vi "Ramp (2).vi"() -> ()   [LabVIEW 2016]
uses:
  controls/Enum.ctl
  <vilib>/rvi/errors/niLvFpgaAdjustHostInterfaceError.vi
  controls/FPGAVIreferenceTypeDef.ctl
  <vilib>/rvi/interface/nirviReadWriteControl/nirviReadWriteControl.xnode
  FPGA Bitfiles/qnmController797_usbRio80MHz_USB7856R80MHz.lvbitx
  <vilib>/rvi/interface/nirviMethod/nirviMethod.xnode
  <vilib>/regexp/Match Regular Expression.xnode
  Course Project/support/Message Queue/Message Queue.lvlib
  <vilib>/rvi/interface/nirviCloseFPGA/nirviCloseFPGA.xnode
  NiFpgaLv.dll
  <vilib>/rvi/errors/niLvFpgaMergeErrorWithErrorCode.vi
  <vilib>/FPGAPlugInAG/USB-7856R/niLvFpga_ReadFifo_USB-7856R.vi
  <vilib>/FPGAPlugInAG/USB-7856R/niLvFpga_Close_USB-7856R.vi
panel:
  in  "Display":T1(array[cluster])
  in  "Palet2":T2={"Save"=FALSE, "Delete"=FALSE, "Show 2"=TRUE}
  in  "Palet1":T2={"Save"=FALSE, "Delete"=FALSE, "Show 2"=TRUE}
  in  "ChannelDisplay2":u16(ring) items=["Height", "AI0 (error)"]
  in  "ChannelDisplay":u16(ring)=1 items=["Height", "AI0 (error)"]
  out "ForceCurves 2":cluster{dbl[], "Decimated Array":dbl[]}[](graph)
  out "ForceCurves":cluster{dbl[], "Decimated Array":dbl[]}[](graph)
  in  "Dec":u16=2 format="%#_3p"
  in  "recordClockDec":u16=100
  in  "SecureTip":T3 {"Sign" items=[">", "<"]; "Secure tip signal" items=["Vert. Deflection (V)", "Horiz. Deflection (V)", "Input 1", "Input 2"]; "Max-min-Tip" format="%#.2p"}
  in  "Curves 2":i32[](listbox)
  in  "Spectroscopy":enum32{"Spectroscopy"}(tab)
  in  "Reenable Feedback":bool=TRUE
  in  "LockSpeed":bool=TRUE
  in  "Direction":bool=TRUE
  in  "Fwd sweep":bool=TRUE
  in  "Parameters":T4={"Start"=-1e-06, "Distance"=1.1e-06, "Points"=1000.0, "Fwd"=5e-07, "Bwd"=5e-07, "Pause"=300.0} {"Pause" format="%#_3fms"; "Bwd" format="%_3pm/s"; "Distance" format="%#.3pm"; "Start" format="%#.3pm"; "Fwd" format="%_3pm/s"}
  out "Ramping?":bool
  in  "Bwd sweep":bool=TRUE
  in  "Output":enum16{"Z"}(ring)
  in  "Channels":i32[](listbox)=[0, 1]
  in  "Actions":T5={"Play"=FALSE, "Stop"=FALSE, "Loop"=FALSE, "Sweeps"=1.0} {"Sweeps" min=1.0 format="%#.0f"}
  in  "CalculateSlope":bool
  out "1/Slope":dbl format="%#_5pm/V"
  out "B":cluster{"Y":dbl, "X":dbl} {"X" format="%#_2p"; "Y" format="%#_2p"}
  out "A":cluster{"Y":dbl, "X":dbl} {"X" format="%#_2p"; "Y" format="%#_2p"}
  in  "Saving":T6={"#"=0, "Name"="", "Path"=path "C:/ForceCurves", "Autosave"=FALSE, "Save"=FALSE} {"#" format="%03.0f"}
  in  "Trigger Source":T7(ring)=enum."Relative Height"
  # "Secure tip"
  # "Spectroscopy"
  # "Trigger"
  # "Ramp"
  # "Cursors"
  # "-"
  # "+"
  # "Saving"
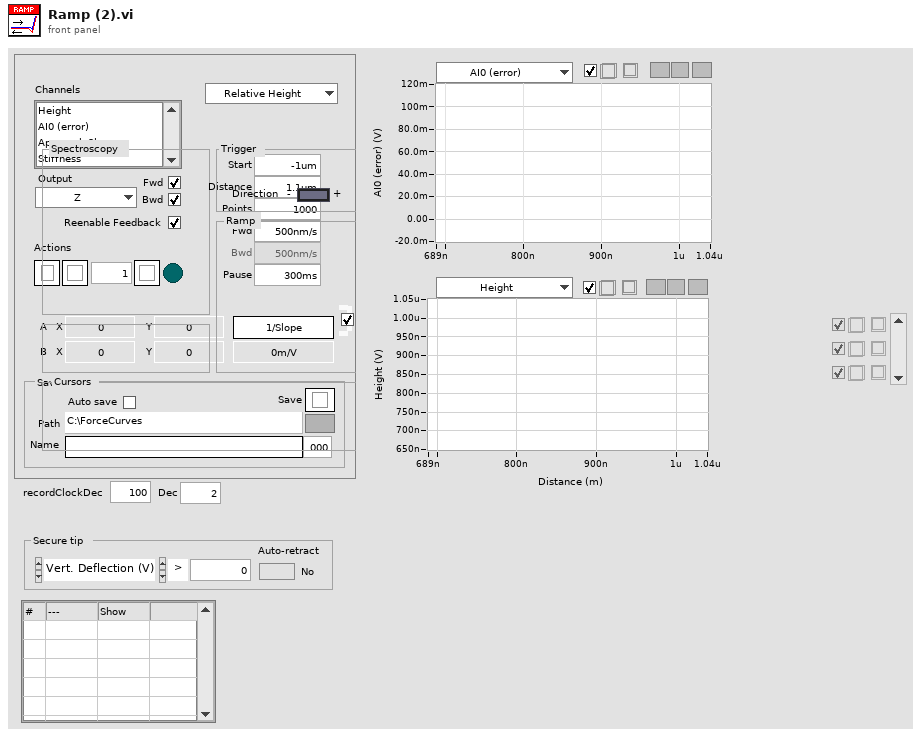
[diagram p1: front panel]
types:
  T1 = cluster{"Save":bool, "Delete":bool, "Show 2":bool}[]
  T2 = cluster{"Save":bool, "Delete":bool, "Show 2":bool}
  T3 = cluster{"Max-min-Tip":dbl, "Secure tip signal":u16, "Sign":u16, "Auto-retract":bool}
  T4 = cluster{"Start":dbl, "Distance":dbl, "Points":dbl, "Fwd":dbl, "Bwd":dbl, "Pause":dbl}
  T5 = cluster{"Play":bool, "Stop":bool, "Loop":bool, "Sweeps":dbl}
  T6 = cluster{"#":i64, "Name":string, "Path":path, "Autosave":bool, "Save":bool}
  T7 = enum16{"Absolute Height", "Process Variable", "External Source", "Relative Height"}
  T8 = typedef "Message Queue.lvlib/All Message Queues.ctl" = cluster{"IU":refnum<queue>}
  T9 = typedef "Enum.ctl" = enum16{"Init", "Read", "Write"}
  T10 = enum32{"Bad", "Idle", "Run top level", "Running"}
  T11 = enum8{"Enabled", "Disabled", "Disabled and Grayed Out"}
  T12 = enum16{"Absolute Height", "Process Variable", "External Source"}
  T13 = cluster{"Range Z":dbl, "Parameters":cluster{"Start":dbl, "Distance":dbl, "Points":dbl, "Fwd":dbl, "Bwd":dbl, "Pause":dbl}, "Trigger Source":enum16{"Absolute Height", "Process Variable", "External Source", "Relative Height"}}
  T14 = enum16{"open", "replace", "create", "open or create", "replace or create", "replace or create with confirmation"}
  T15 = cluster{"calibName":string[], "calibParameters":cluster{"Sensitivity":cluster{"Sens X":dbl, "Sens Y":dbl, "Sens Z":dbl}, "Range":cluster{"Range X":dbl, "Range Y":dbl, "Range Z":dbl}, "HV gain":cluster{"HV gain X":dbl, "HV gain Y":dbl, "HV gain Z":dbl}}[], "calibIndex":i32}
  T16 = cluster{"Sensitivity":cluster{"Sens X":dbl, "Sens Y":dbl, "Sens Z":dbl}, "Range":cluster{"Range X":dbl, "Range Y":dbl, "Range Z":dbl}, "HV gain":cluster{"HV gain X":dbl, "HV gain Y":dbl, "HV gain Z":dbl}}[]
  T17 = cluster{"Sensitivity":cluster{"Sens X":dbl, "Sens Y":dbl, "Sens Z":dbl}, "Range":cluster{"Range X":dbl, "Range Y":dbl, "Range Z":dbl}, "HV gain":cluster{"HV gain X":dbl, "HV gain Y":dbl, "HV gain Z":dbl}}
  T18 = typedef "FPGAVIreferenceTypeDef.ctl" = refnum<k20>
  T19 = typedef "FPGAVIreferenceTypeDefScanEngine.ctl" = refnum<k20>
  T20 = cluster{"enableManualMotion":bool, "doMove":bool, "integratorTarget":fxp<+/-,22,2>, "clocks":cluster{"inverseDecimation":fxp<+,22,0>, "decimation":u16, "waveSize":u16, "pixelDecimation":u16}}
  T21 = cluster{"rmp.p.resetStartPos":bool, "rmp.p.resetEndPos":bool}
  T22 = cluster{"rmp.p.downRate":fxp<+/-,22,-10>, "rmp.p.upRate":fxp<+/-,22,-10>, "rmp.p.startPos":fxp<+/-,24,2>, "rmp.p.clockDec":u16, "rmp.p.recordClockDec":u16, "rmp.p.enableHDTPointRecord":bool, "rmp.p.pull":bool}
  T23 = cluster{"rmp.triggerSource":u8, "rmp.p.triggerPositive":bool, "rmp.p.triggerLevel":fxp<+/-,24,16>}
  T24 = typedef "LVPointDoubleTypeDef.ctl" = cluster{"Cursor X":dbl, "Cursor Y":dbl}
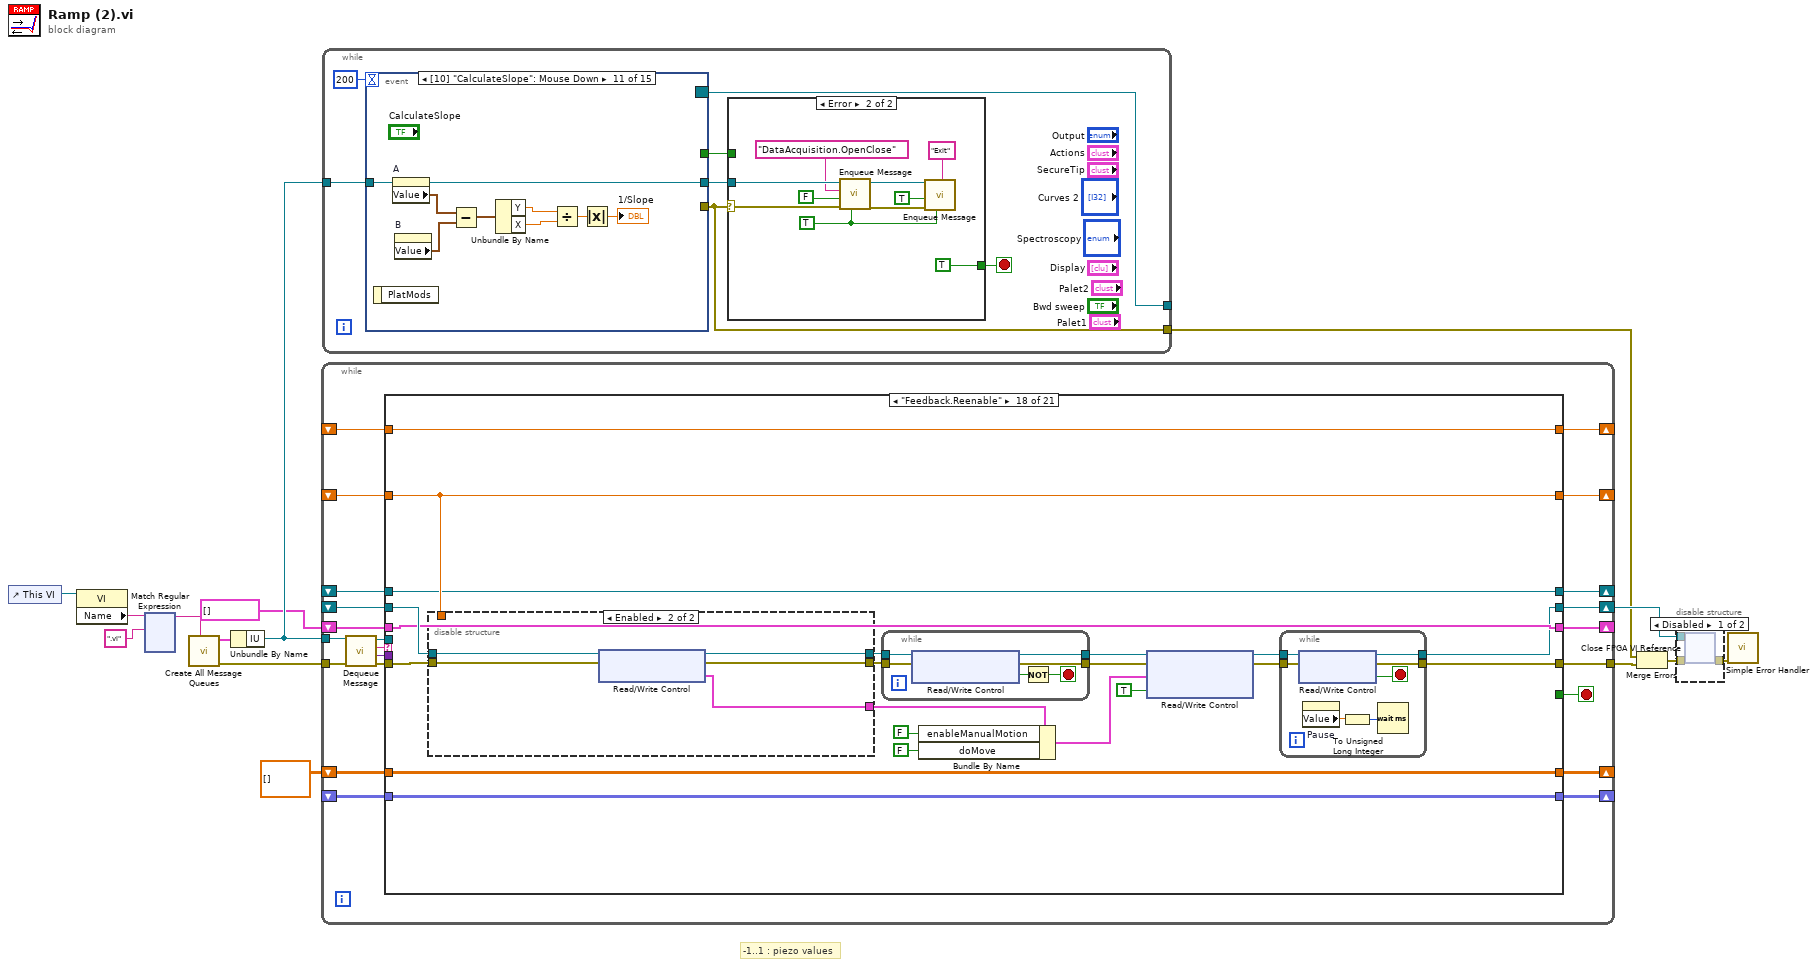
[diagram p0: block diagram]
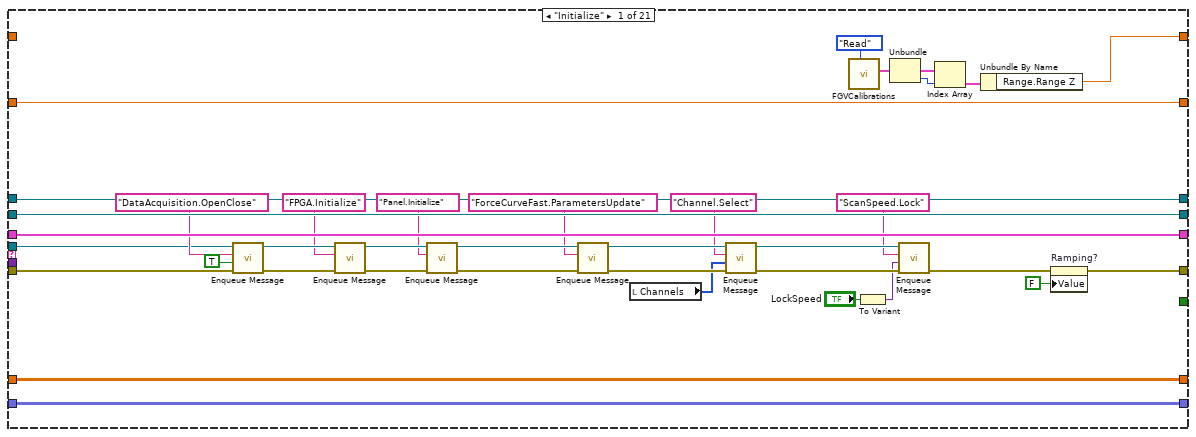
[diagram p3: hidden frame]
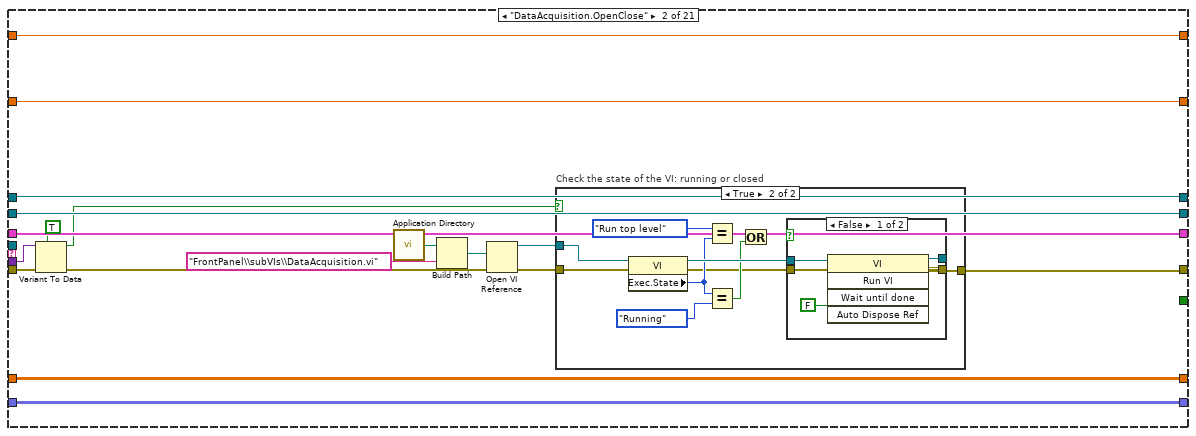
[diagram p4: hidden frame]
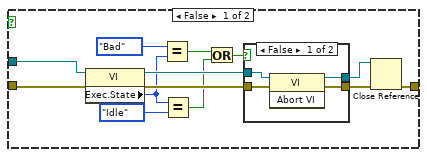
[diagram p5: hidden frame]
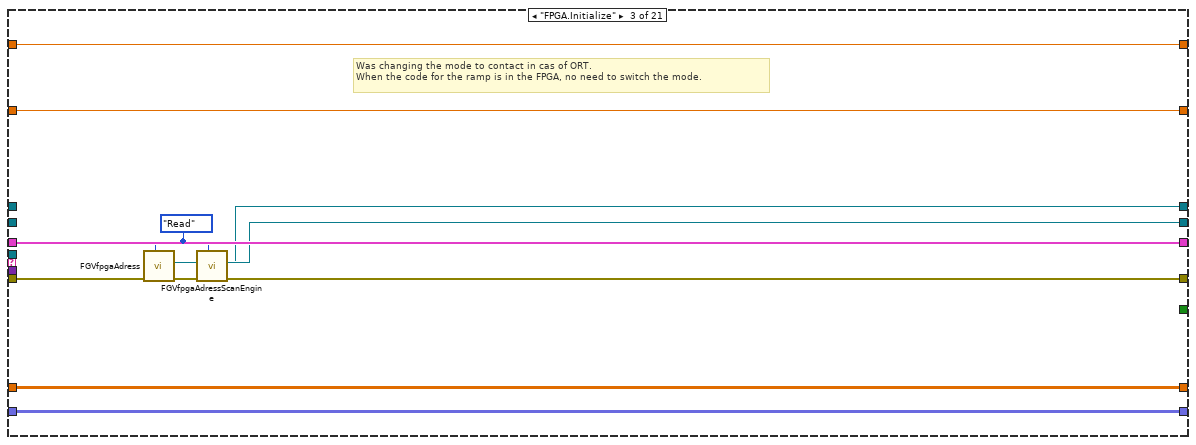
[diagram p8: hidden frame]
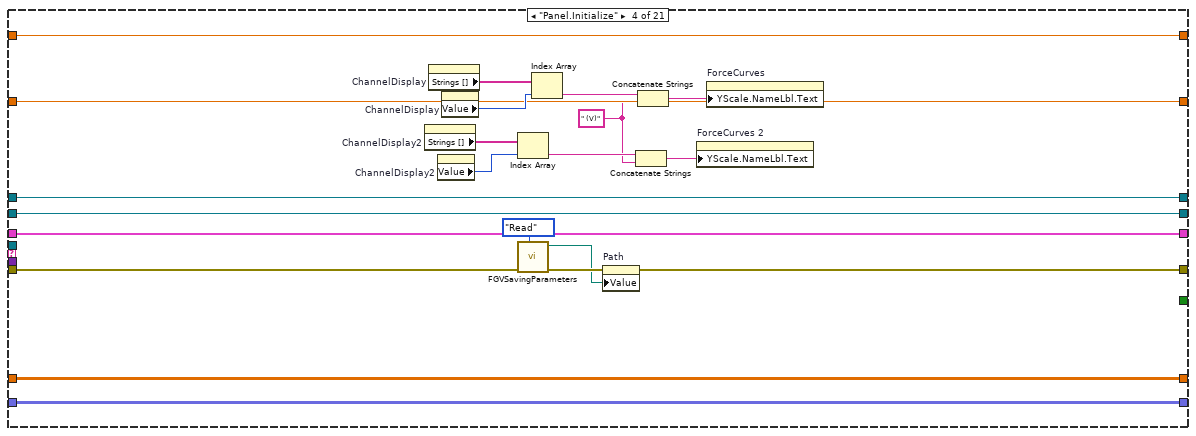
[diagram p9: hidden frame]
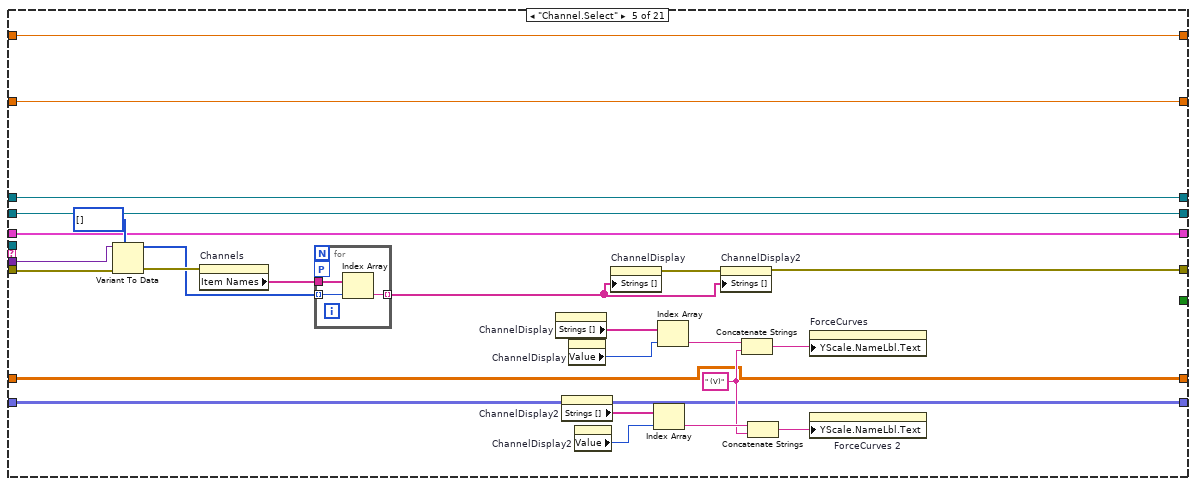
[diagram p10: hidden frame]
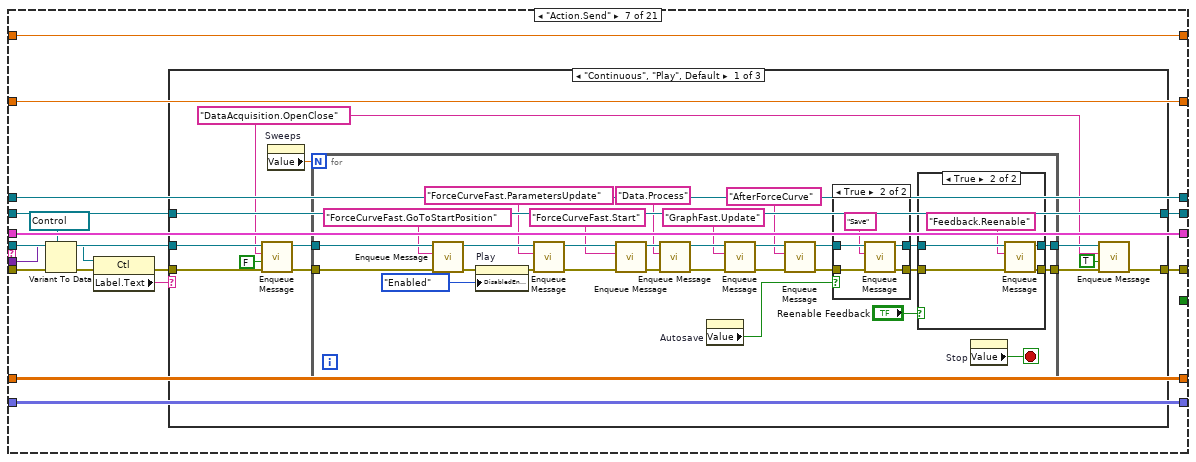
[diagram p12: hidden frame]
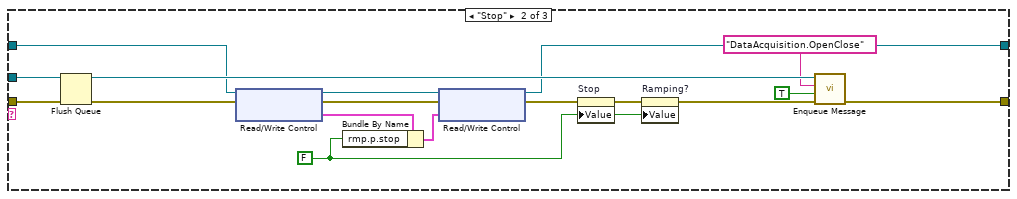
[diagram p15: hidden frame]
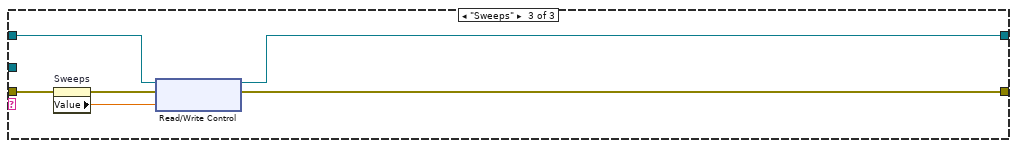
[diagram p16: hidden frame]
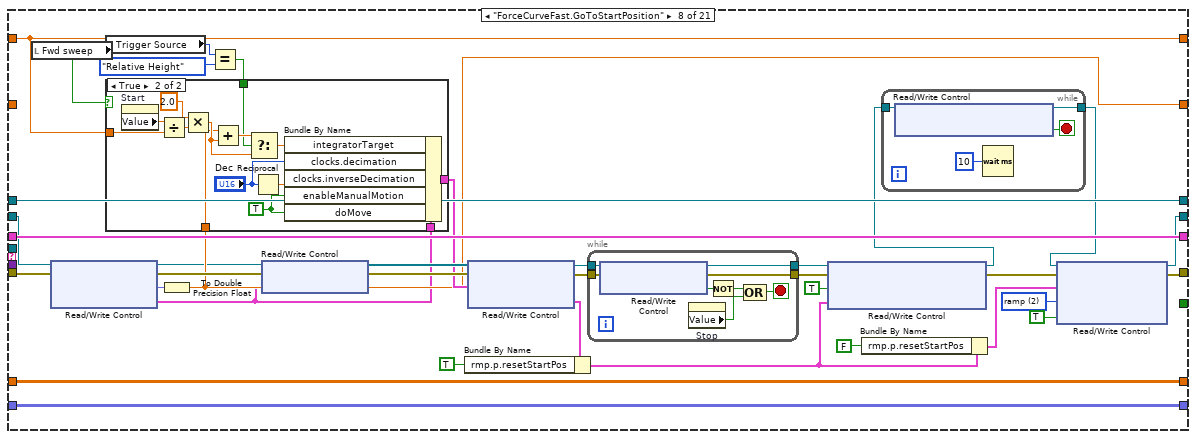
[diagram p17: hidden frame]
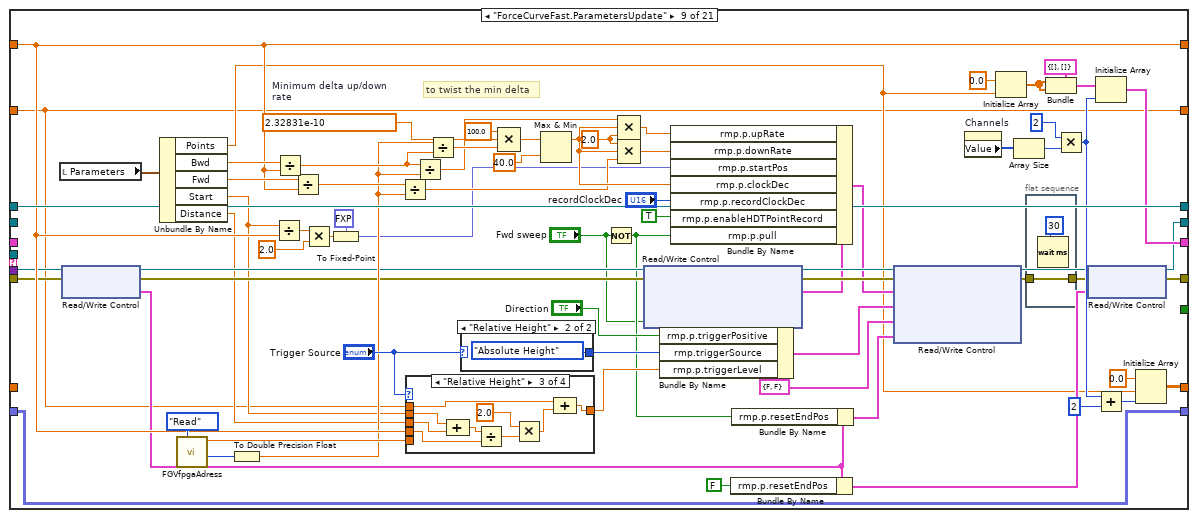
[diagram p19: hidden frame]
diagram:
  # "-1..1 : piezo values"
  n1 = control-ref of="This VI"() -> (w4:refnum<vi>)
  n2 = property class="VI"(reference=w4) -> ("Name"=w3:string)  [unwired: 1 in, 2 out]
  n3 = xnode "Match Regular Expression"("input string"=w3, "regular expression"=".vi") -> ("before match"=w1:string)  [unwired: 4 in, 4 out]
  n4 = call "Create All Message Queues.vi"("QueueName"=w1) -> ("ErrorOut"=w9:errorcluster, "MessageQueueOut"=w14:T8)  [unwired: 9 in]
  n5 = Unbundle By Name(w14) -> ("IU"=w8:refnum<queue>)
  n6 = while {
    shift-right: [w32] -> w10
    shift-left: _ -> [w31]
    tunnel: [w30] -> w11
    tunnel: w9 -> [w28]
    tunnel: w8 -> [w27]
    shift-right: [w25] -> _
    shift-left: _ -> [w26]
    shift-right: [w24] -> _
    shift-left: _ -> [w23]
    shift-right: [w22] -> _
    shift-left: _ -> [w21]
    shift-right: [w20] -> _
    shift-left: _ -> [w19]
    shift-right: [w17] -> _
    shift-left: cluster{dbl[], "Decimated Array":dbl[]}[] [] ("GraphOut") -> [w18]
    shift-right: [w15] -> _
    shift-left: dbl[][] [] ("SaveArrayOut") -> [w16]
    stop <- w36 stop-if-true
    n7 = call "Dequeue Message.vi"("entrée d'erreur (pas d'erreur)"=w28, "File d'attente de messages"=w27) -> ("sortie d'erreur"=w35:errorcluster, "Données de message"=w34:variant, "Message"=w29:string, "File d'attente de message dup."=w33:refnum<queue>)  [unwired: 6 in]
    n8 = case shown="\"Feedback.Reenable\"" w29 {
      selector: w29 -> [_ _ _ _ _ _ _ _ _ _ _ _ _ _ _ _ _ _ _ _ w902]
      tunnel: w33 -> [w44 _ _ _ _ _ w212 _ _ _ _ _ _ _ _ _ w767 _ _ _ _]
      tunnel: w35 -> [w46 w83 w137 w148 w179 w195 w205 w319 w373 w487 w517 w585 w630 w645 w662 w724 w764 w782 w858 w888 _]
      tunnel: [w56 w75 w134 w146 w180 w195 w202 w312 w361 errorcluster {"status"=FALSE, "code"=0, "source"=""} ("error out") w520 w570 w630 w637 w663 w708 w763 w768 w857 w887 w900] -> w30
      tunnel: [_ _ _ _ _ _ _ _ _ _ _ _ _ _ _ _ TRUE _ _ _ _] -> w36
      tunnel: w34 -> [_ w82 _ _ w177 _ w210 _ _ _ _ _ _ w644 w660 _ _ _ w856 _ _]
      tunnel: [w68 w89 w135 w156 w184 w194 w200 w313 w362 w452 w519 w583 w588 w652 w667 w723 w762 w769 w860 w891 w898] -> w32
      tunnel: w31 -> [w68 w89 _ w156 w184 w194 w206 w320 w371 w461 w516 w583 w588 w652 w667 w723 w762 w783 w860 w891 w898]
      tunnel: w26 -> [_ w88 w136 w155 w183 w193 w201 w317 w397 w484 w515 w574 w629 w651 w665 w722 w761 w788 w859 w890 w897]
      tunnel: [w61 w88 w136 w155 w183 w193 w201 w317 w397 w484 w515 w574 w629 w651 w665 w722 w761 w788 w859 w890 w897] -> w25
      tunnel: [w55 w87 w133 w150 w182 w192 w199 w298 w354 w485 w514 w571 w628 w650 w666 w711 w760 w780 w864 w889 w896] -> w24
      tunnel: w23 -> [w55 w87 w133 w150 w182 w192 w199 _ w354 w485 w514 w571 w628 w650 w666 w711 w760 w780 w864 w889 w896]
      tunnel: [w49 w86 w132 w140 w163 w191 w198 w311 w395 w471 w524 w582 w627 w649 w658 w730 w759 w777 w834 w885 w895] -> w22
      tunnel: w21 -> [w49 w86 w132 w140 w163 w191 w198 w311 w395 _ w524 w582 w627 w649 w658 w730 w759 w777 w834 w885 w895]
      tunnel: [w71 w85 w129 w139 w162 w190 w197 w323 w426 w462 w523 w584 w626 w648 w655 w701 w758 w776 w833 w884 w894] -> w20
      tunnel: w19 -> [w71 w85 _ w139 w162 w190 w197 w323 w426 w462 w523 w584 w626 w648 w655 w701 w758 w776 w833 w884 w894]
      tunnel: w18 -> [w73 w91 w138 w159 w160 w188 w211 w324 _ w488 w522 w576 w617 w647 w653 w726 w756 w774 w861 w882 w892]
      tunnel: [w73 w91 w138 w159 w160 w188 w211 w324 w385 w488 w522 w575 w617 w647 w653 w726 w756 w774 w861 w882 w892] -> w17
      tunnel: w16 -> [w43 w74 w128 w158 w161 w189 w196 w305 _ w486 w521 w573 w600 w646 w654 w728 w757 w775 w862 w883 w893]
      tunnel: [w43 w74 w128 w158 w161 w189 w196 w305 w382 w486 w521 w572 w600 w646 w654 w728 w757 w775 w862 w883 w893] -> w15
      frame "Initialize" {
        n9 = call "Enqueue Message.vi"("error in"=w46, "Data"=TRUE, "Message"="DataAcquisition.OpenClose", "Queue"=w44) -> ("error out"=w47:errorcluster, "Queue dup."=w72:refnum<queue>)  [unwired: 6 in]
        n10 = call "Enqueue Message.vi"("error in"=w47, "Message"="FPGA.Initialize", "Queue"=w72) -> ("error out"=w59:errorcluster, "Queue dup."=w58:refnum<queue>)  [unwired: 7 in]
        n11 = call "Enqueue Message.vi"("error in"=w59, "Message"="Panel.Initialize", "Queue"=w58) -> ("error out"=w51:errorcluster, "Queue dup."=w52:refnum<queue>)  [unwired: 7 in]
        n12 = call "Enqueue Message.vi"("error in"=w51, "Message"="ForceCurveFast.ParametersUpdate", "Queue"=w52) -> ("error out"=w70:errorcluster, "Queue dup."=w69:refnum<queue>)  [unwired: 7 in]
        n13 = local read "Channels"() -> (w53:i32[])
        n14 = call "Enqueue Message.vi"("error in"=w70, "Data"=w53, "Message"="Channel.Select", "Queue"=w69) -> ("error out"=w42:errorcluster, "Queue dup."=w40:refnum<queue>)  [unwired: 6 in]
        n15 = call "FGVCalibrations.vi"("Enum"=Enum."Read") -> ("calibOut"=w65:T15)  [unwired: 9 in, 1 out]
        n16 = To Variant(anything="LockSpeed") -> (Variant=w37:variant)
        n17 = Unbundle(w65) -> ("calibParameters"=w63:T16, "calibIndex"=w62:i32)  [unwired: 1 out]
        n18 = call "Enqueue Message.vi"("error in"=w42, "Data"=w37, "Message"="ScanSpeed.Lock", "Queue"=w40) -> ("error out"=w41:errorcluster)  [unwired: 6 in, 1 out]
        n19 = Index Array(array=w63, index=w62) -> (element=w66:T17)
        n20 = Unbundle By Name(w66) -> ("Range.Range Z"=w61:dbl)
        n21 = property on="Ramping?" class="Bool (strict)"(error in=w41, "Value"=FALSE ("Ramping?")) -> (error out=w56:errorcluster)  [unwired: 1 in, 1 out]
      }
      frame "DataAcquisition.OpenClose" {
        n22 = Variant To Data(error in=w83, type=TRUE, Variant=w82) -> (data=w76:bool, error out=w90:errorcluster)
        n23 = call <vilib>:"Application Directory.vi"() -> ("Application Directory"=w78:path)
        n24 = Build Path(base path=w78, name or relative path="FrontPanel\\subVIs\\DataAcquisition.vi") -> (appended path=w79:path)
        n25 = Open VI Reference(vi path=w79, error in (no error)=w90) -> (vi reference=w77:refnum<vi>, error out=w80:errorcluster)  [unwired: 4 in]
        n26 = case "Check the state of the VI: running or closed" shown="True" w76 {
          tunnel: w80 -> [w102 w111]
          tunnel: w77 -> [w95 w120]
          tunnel: [w92 w119] -> w75
          frame False {
            n27 = property class="VI"(reference=w95) -> (reference out=w103:refnum<vi>, "Exec.State"=w97:T10)  [unwired: 1 in, 1 out]
            n28 = Equal?(x=T10."Bad" ("Execution:State"), y=w97) -> (x = y?=w99:bool)
            n29 = Equal?(x=w97, y=T10."Idle" ("Execution:State")) -> (x = y?=w100:bool)
            n30 = Or(x=w99, y=w100) -> (x .or. y?=w101:bool)
            n31 = case shown="False" w101 {
              tunnel: [w107 w109] -> w94
              tunnel: [w106 w108] -> w93
              tunnel: w102 -> [w105 w108]
              tunnel: w103 -> [w104 w109]
              frame False {
                n32 = invoke class="VI" method="Abort VI"(reference=w104, error in=w105) -> (reference out=w107:refnum<vi>, error out=w106:errorcluster)  [unwired: 1 in, 1 out]
              }
              frame True {
              }
            }
            n33 = Close Reference(reference=w94, error in (no error)=w93) -> (error out=w92:errorcluster)
          }
          frame True {
            n34 = property class="VI"(reference=w120, error in=w111) -> (reference out=w118:refnum<vi>, error out=w110:errorcluster, "Exec.State"=w116:T10)
            n35 = Equal?(x=T10."Run top level" ("Execution:State"), y=w116) -> (x = y?=w114:bool)
            n36 = Equal?(x=w116, y=T10."Running" ("Execution:State")) -> (x = y?=w113:bool)
            n37 = Or(x=w114, y=w113) -> (x .or. y?=w112:bool)
            n38 = case shown="False" w112 {
              tunnel: [w122 w127] -> _
              tunnel: [w121 w126] -> w119
              tunnel: w110 -> [w123 w126]
              tunnel: w118 -> [w124 w127]
              frame False {
                n39 = invoke class="VI" method="Run VI"(reference=w124, error in=w123, "Wait until done"=FALSE ("Wait Until Done")) -> (reference out=w122:refnum<vi>, error out=w121:errorcluster)  [unwired: 2 in, 3 out]
              }
              frame True {
              }
            }
          }
        }
      }
      frame "FPGA.Initialize" {
        w130 = Enum."Read" ("Enum")
        # "Was changing the mode to contact in cas of ORT.\nWhen the code for the ramp is in the FPGA, no need to switch the mode."
        n40 = call "FGVfpgaAdress.vi"("Enum"=w130, "error in"=w137) -> ("error out"=w131:errorcluster, "FPGA VI Reference Out"=w135:T18)  [unwired: 4 in, 4 out]
        n41 = call "FGVfpgaAdressScanEngine.vi"("Enum"=w130, "error in"=w131) -> ("error out"=w134:errorcluster, "FPGA.SEout"=w129:T19)  [unwired: 5 in, 3 out]
      }
      frame "Panel.Initialize" {
        w141 = " (V)" ("Y Scale.Unit Label.Text")
        n42 = property on="ChannelDisplay2" class="Ring (strict)"() -> ("Strings []"=w153:string[])  [unwired: 2 in, 2 out]
        n43 = property on="ChannelDisplay" class="Ring (strict)"() -> ("Strings []"=w154:string[])  [unwired: 2 in, 2 out]
        n44 = property on="ChannelDisplay2" class="Ring (strict)"() -> ("Value"=w152:u16)  [unwired: 2 in, 2 out]
        n45 = property on="ChannelDisplay" class="Ring (strict)"() -> ("Value"=w151:u16)  [unwired: 2 in, 2 out]
        n46 = Index Array(array=w153, index=w152) -> (element=w144:string)
        n47 = call "FGVSavingParameters.vi"("Enum"=Enum."Read", "error in"=w148) -> ("error out"=w157:errorcluster, "pathOut"=w147:path)  [unwired: 6 in, 2 out]
        n48 = Index Array(array=w154, index=w151) -> (element=w145:string)
        n49 = property on="Path" class="Path"(error in=w157, "Value"=w147) -> (error out=w146:errorcluster)  [unwired: 1 in, 1 out]
        n50 = Concatenate Strings(w144, w141) -> (w143:string)
        n51 = Concatenate Strings(w145, w141) -> (w142:string)
        n52 = property on="ForceCurves 2" class="XYGraph (strict)"("YScale.NameLbl.Text"=w143) -> ()  [unwired: 2 in, 2 out]
        n53 = property on="ForceCurves" class="XYGraph (strict)"("YScale.NameLbl.Text"=w142) -> ()  [unwired: 2 in, 2 out]
      }
      frame "Channel.Select" {
        w164 = " (V)" ("Y Scale.Unit Label.Text")
        n54 = Variant To Data(error in=w179, type=i32[] [] ("NewVal"), Variant=w177) -> (data=w174:i32[], error out=w176:errorcluster)
        n55 = property on="Channels" class="LstBox (strict)"(error in=w176) -> ("Item Names"=w175:string[])  [unwired: 1 in, 2 out]
        n56 = for {
          tunnel: w175 -> [w187]
          tunnel: w174 -> [w186] mode=indexing
          tunnel: [w185] -> w173 mode=indexing
          workers-P: _ -> [_]
          n57 = Index Array(array=w187, index=w186) -> (element=w185:string)
        }
        n58 = property on="ChannelDisplay" class="Ring (strict)"() -> ("Strings []"=w172:string[])  [unwired: 2 in, 2 out]
        n59 = property on="ChannelDisplay2" class="Ring (strict)"() -> ("Strings []"=w171:string[])  [unwired: 2 in, 2 out]
        n60 = property on="ChannelDisplay" class="Ring (strict)"() -> ("Value"=w169:u16)  [unwired: 2 in, 2 out]
        n61 = property on="ChannelDisplay2" class="Ring (strict)"() -> ("Value"=w170:u16)  [unwired: 2 in, 2 out]
        n62 = property on="ChannelDisplay" class="Ring (strict)"("Strings []"=w173) -> (error out=w181:errorcluster)  [unwired: 2 in, 1 out]
        n63 = Index Array(array=w171, index=w170) -> (element=w168:string)
        n64 = Index Array(array=w172, index=w169) -> (element=w167:string)
        n65 = property on="ChannelDisplay2" class="Ring (strict)"(error in=w181, "Strings []"=w173) -> (error out=w180:errorcluster)  [unwired: 1 in, 1 out]
        n66 = Concatenate Strings(w167, w164) -> (w166:string)
        n67 = Concatenate Strings(w168, w164) -> (w165:string)
        n68 = property on="ForceCurves" class="XYGraph (strict)"("YScale.NameLbl.Text"=w166) -> ()  [unwired: 2 in, 2 out]
        n69 = property on="ForceCurves 2" class="XYGraph (strict)"("YScale.NameLbl.Text"=w165) -> ()  [unwired: 2 in, 2 out]
      }
      frame "Channel.Display" {
      }
      frame "Action.Send" {
        n70 = Variant To Data(error in=w205, type=refnum<vi> refnum ("CtlRef"), Variant=w210) -> (data=w208:refnum<vi>, error out=w207:errorcluster)
        n71 = property class="Ctl"(reference=w208, error in=w207) -> (error out=w203:errorcluster, "Label.Text"=w204:string)  [unwired: 1 out]
        n72 = case shown="\"Continuous\", \"Play\", Default" w204 {
          tunnel: w206 -> [w223 w276 w290]
          tunnel: w203 -> [w215 w281 w288]
          tunnel: [w219 w268 w286] -> w202
          tunnel: [w223 w280 w285] -> w200
          tunnel: w212 -> [w217 w282 _]
          frame "Continuous", "Play", Default {
            w213 = "DataAcquisition.OpenClose" ("Message")
            n73 = call "Enqueue Message.vi"("error in"=w215, "Data"=FALSE, "Message"=w213, "Queue"=w217) -> ("error out"=w214:errorcluster, "Queue dup."=w216:refnum<queue>)  [unwired: 6 in]
            n74 = property on="Sweeps" class="DigNum (strict)"() -> ("Value"=w222:dbl)  [unwired: 2 in, 2 out]
            n75 = for {
              N: w222 -> [_]
              tunnel: w216 -> [w253]
              tunnel: w214 -> [w228]
              tunnel: [w251] -> w220
              tunnel: [w225] -> w224
              stop <- w250 stop-if-true
              n76 = call "Enqueue Message.vi"("error in"=w228, "Message"="ForceCurveFast.GoToStartPosition", "Queue"=w253) -> ("error out"=w246:errorcluster, "Queue dup."=w244:refnum<queue>)  [unwired: 7 in]
              n77 = property on="Play" class="Bool (strict)"(error in=w246, "DisabledEnum"=T11."Enabled" ("Disabled")) -> (error out=w243:errorcluster)  [unwired: 1 in, 1 out]
              n78 = call "Enqueue Message.vi"("error in"=w243, "Message"="ForceCurveFast.ParametersUpdate", "Queue"=w244) -> ("error out"=w240:errorcluster, "Queue dup."=w241:refnum<queue>)  [unwired: 7 in]
              n79 = call "Enqueue Message.vi"("error in"=w240, "Message"="ForceCurveFast.Start", "Queue"=w241) -> ("error out"=w235:errorcluster, "Queue dup."=w248:refnum<queue>)  [unwired: 7 in]
              n80 = call "Enqueue Message.vi"("error in"=w235, "Message"="Data.Process", "Queue"=w248) -> ("error out"=w234:errorcluster, "Queue dup."=w249:refnum<queue>)  [unwired: 7 in]
              n81 = property on="Autosave" class="Bool (strict)"() -> ("Value"=w231:bool)  [unwired: 2 in, 2 out]
              n82 = call "Enqueue Message.vi"("error in"=w234, "Message"="GraphFast.Update", "Queue"=w249) -> ("error out"=w229:errorcluster, "Queue dup."=w252:refnum<queue>)  [unwired: 7 in]
              n83 = call "Enqueue Message.vi"("error in"=w229, "Message"="AfterForceCurve", "Queue"=w252) -> ("error out"=w226:errorcluster, "Queue dup."=w227:refnum<queue>)  [unwired: 7 in]
              n84 = case shown="True" w231 {
                tunnel: w226 -> [w254 w260]
                tunnel: [w254 w259] -> w233
                tunnel: w227 -> [w255 w258]
                tunnel: [w255 w257] -> w232
                frame False {
                }
                frame True {
                  n85 = call "Enqueue Message.vi"("error in"=w260, "Message"="Save", "Queue"=w258) -> ("error out"=w259:errorcluster, "Queue dup."=w257:refnum<queue>)  [unwired: 7 in]
                }
              }
              n86 = case shown="True" "Reenable Feedback" {
                tunnel: w233 -> [w262 w265]
                tunnel: [w262 w264] -> w251
                tunnel: w232 -> [w261 w267]
                tunnel: [w261 w263] -> w225
                frame False {
                }
                frame True {
                  n87 = call "Enqueue Message.vi"("error in"=w265, "Message"="Feedback.Reenable", "Queue"=w267) -> ("error out"=w264:errorcluster, "Queue dup."=w263:refnum<queue>)  [unwired: 7 in]
                }
              }
              n88 = property on="Stop" class="Bool (strict)"() -> ("Value"=w250:bool)  [unwired: 2 in, 2 out]
            }
            n89 = call "Enqueue Message.vi"("error in"=w220, "Data"=TRUE, "Message"=w213, "Queue"=w224) -> ("error out"=w219:errorcluster)  [unwired: 6 in, 1 out]
          }
          frame "Stop" {
            w272 = FALSE ("Value")
            n90 = Flush Queue(queue=w282, error in (no error)=w281) -> (queue out=w284:refnum<queue>, error out=w275:errorcluster)  [unwired: 1 out]
            n91 = xnode "Read/Write Control"("FPGA VI Reference In"=w276, "error in"=w275) -> ("FPGA VI Reference Out"=w277:T18, "error out"=w278:errorcluster, "rmp.p.action"=w274:cluster{"rmp.p.start":bool, "rmp.p.stop":bool})
            n92 = Bundle By Name(cluster=w274, "rmp.p.stop"=w272) -> (w273:cluster{"rmp.p.start":bool, "rmp.p.stop":bool})
            n93 = xnode "Read/Write Control"("FPGA VI Reference In"=w277, "error in"=w278, "rmp.p.action"=w273) -> ("FPGA VI Reference Out"=w280:T18, "error out"=w279:errorcluster)
            n94 = property on="Stop" class="Bool (strict)"(error in=w279, "Value"=w272) -> (error out=w283:errorcluster)  [unwired: 1 in, 1 out]
            n95 = property on="Ramping?" class="Bool (strict)"(error in=w283, "Value"=w272) -> (error out=w269:errorcluster)  [unwired: 1 in, 1 out]
            n96 = call "Enqueue Message.vi"("error in"=w269, "Data"=TRUE, "Message"="DataAcquisition.OpenClose", "Queue"=w284) -> ("error out"=w268:errorcluster)  [unwired: 6 in, 1 out]
          }
          frame "Sweeps" {
            n97 = property on="Sweeps" class="DigNum (strict)"(error in=w288) -> (error out=w287:errorcluster, "Value"=w289:dbl)  [unwired: 1 in, 1 out]
            n98 = xnode "Read/Write Control"("FPGA VI Reference In"=w290, "error in"=w287, "lwr.p.avgCnt"=w289) -> ("FPGA VI Reference Out"=w285:T18, "error out"=w286:errorcluster)
          }
        }
      }
      frame "ForceCurveFast.GoToStartPosition" {
        w314 = u8 2 items=["process Variable", "SICM", "ramp"] ("flt.i.bypassSource")
        n99 = local read "Fwd sweep"() -> (w299:bool)
        n100 = xnode "Read/Write Control"("FPGA VI Reference In"=w320, "error in"=w319) -> ("FPGA VI Reference Out"=w293:T18, "error out"=w325:errorcluster, "fb.o.height"=w297:fxp<+/-,31,4>, "fb.mot.p.params"=w291:T20)
        n101 = local read "Trigger Source"() -> (w296:T7)
        n102 = To Double Precision Float(number=w297) -> (double precision float=w298:dbl)
        n103 = Equal?(x=w296, y=T7."Relative Height" ("Trigger Source")) -> (x = y?=w295:bool)
        n104 = case shown="True" w299 {
          tunnel: w291 -> [w327 w339]
          tunnel: [w327 w338] -> w318
          tunnel: w317 -> [_ w337]
          tunnel: w298 -> [_ w330]
          tunnel: w295 -> [_ w328]
          frame False {
          }
          frame True {
            w341 = TRUE ("doMove")
            n105 = property on="Start" class="DigNum (strict)"() -> ("Value"=w340:dbl)  [unwired: 2 in, 2 out]
            n106 = Divide(x=w340, y=w337) -> (x/y=w335:dbl)
            n107 = Multiply(x=2.0 ("y"), y=w335) -> (x*y=w332:dbl)
            n108 = Add(x=w330, y=w332) -> (x+y=w333:dbl)
            n109 = Select(t=w333, s=w328, f=w332) -> (s? t:f=w331:dbl)
            n110 = Reciprocal(x="Dec") -> (1/x=w336:dbl)
            n111 = Bundle By Name(cluster=w339, "integratorTarget"=w331, "clocks.decimation"="Dec", "clocks.inverseDecimation"=w336, "enableManualMotion"=w341, "doMove"=w341) -> (w338:T20)
          }
        }
        n112 = xnode "Read/Write Control"("FPGA VI Reference In"=w293, "error in"=w325, "fb.mot.p.params"=w291) -> ("FPGA VI Reference Out"=w292:T18, "error out"=w326:errorcluster)
        n113 = xnode "Read/Write Control"("FPGA VI Reference In"=w292, "error in"=w326, "fb.mot.p.params"=w318) -> ("FPGA VI Reference Out"=w321:T18, "error out"=w322:errorcluster, "rmp.p.reset"=w309:T21)
        n114 = Bundle By Name(cluster=w309, "rmp.p.resetStartPos"=TRUE) -> (w307:T21)
        n115 = while {
          tunnel: w322 -> [w353]
          tunnel: [w352] -> w316
          tunnel: [w351] -> w315
          tunnel: w321 -> [w350]
          stop <- w346 stop-if-true
          n116 = xnode "Read/Write Control"("FPGA VI Reference In"=w350, "error in"=w353) -> ("FPGA VI Reference Out"=w352:T18, "error out"=w351:errorcluster, "fb.mot.s.running"=w347:bool)
          n117 = property on="Stop" class="Bool (strict)"() -> ("Value"=w348:bool)  [unwired: 2 in, 2 out]
          n118 = Not(x=w347) -> (.not. x?=w349:bool)
          n119 = Compound Arithmetic op=OR(w349, w348) -> (w346:bool)
        }
        n120 = xnode "Read/Write Control"("FPGA VI Reference In"=w316, "error in"=w315, "rmp.p.useIntHeightAsStart"=TRUE, "rmp.p.reset"=w307) -> ("FPGA VI Reference Out"=w300:T18, "error out"=w303:errorcluster)
        n121 = Bundle By Name(cluster=w307, "rmp.p.resetStartPos"=FALSE) -> (w304:T21)
        n122 = while {
          tunnel: w300 -> [w345]
          tunnel: [w344] -> w302
          stop <- w343 stop-if-true
          n123 = xnode "Read/Write Control"("FPGA VI Reference In"=w345) -> ("FPGA VI Reference Out"=w344:T18, "rmp.p.useIntHeightAsStart"=w343:bool)  [unwired: 1 in, 1 out]
          n124 = Wait (ms)(milliseconds to wait=u32 10) -> ()  [unwired: 1 out]
        }
        n125 = xnode "Read/Write Control"("FPGA VI Reference In"=w302, "error in"=w303, "rmp.p.reset"=w304, "flt.i.bypassSource"=w314, "flt.bypassPI"=TRUE) -> ("FPGA VI Reference Out"=w313:T18, "error out"=w312:errorcluster)
      }
      frame "ForceCurveFast.ParametersUpdate" {
        w378 = 2.0
        w410 = 2.32831e-10  # Minimum delta up/down rate
        # "to twist the min delta"
        n126 = local read "Parameters"() -> (w413:T4)
        n127 = xnode "Read/Write Control"("FPGA VI Reference In"=w371, "error in"=w373) -> ("FPGA VI Reference Out"=w370:T18, "error out"=w372:errorcluster, "rmp.p.reset"=w367:T21)
        n128 = Unbundle By Name(w413) -> ("Points"=w359:dbl, "Bwd"=w399:dbl, "Fwd"=w398:dbl, "Start"=w365:dbl, "Distance"=w355:dbl)
        n129 = call "FGVfpgaAdress.vi"("Enum"=Enum."Read") -> ("baseClockOut"=w402:u32, "voltageRange(+/-)Out"=w412:dbl)  [unwired: 5 in, 4 out]
        n130 = To Double Precision Float(number=w402) -> (double precision float=w377:dbl)
        n131 = Divide(x=w365, y=w397) -> (x/y=w420:dbl)
        n132 = Divide(x=w399, y=w397) -> (x/y=w403:dbl)
        n133 = Divide(x=w398, y=w397) -> (x/y=w401:dbl)
        n134 = Multiply(x=w420, y=2.0) -> (x*y=w417:dbl)
        n135 = To Fixed-Point(fixed-point type=fxp<+/-,24,2> 0.0 ("rmp.p.startPos"), number=w417) -> (fixed-point=w364:fxp<+/-,24,2>)
        n136 = Divide(x=w401, y=w377) -> (x/y=w400:dbl)
        n137 = case shown="\"Relative Height\"" "Trigger Source" {
          tunnel: w397 -> [_ w440 w449 _]
          tunnel: [w434 w437 w441 w450] -> w416
          tunnel: w412 -> [w432 _ _ _]
          tunnel: w355 -> [w431 w436 w445 w450]
          tunnel: w365 -> [_ _ w446 _]
          tunnel: w354 -> [_ _ w443 _]
          frame "Process Variable", Default {
            n138 = Divide(x=w431, y=w432) -> (x/y=w435:dbl)
            n139 = Multiply(x=32767.0, y=w435) -> (x*y=w434:dbl)
          }
          frame "Absolute Height" {
            n140 = Divide(x=w436, y=w440) -> (x/y=w438:dbl)
            n141 = Multiply(x=2.0, y=w438) -> (x*y=w437:dbl)
          }
          frame "Relative Height" {
            n142 = Compound Arithmetic op=ADD(w446, w445) -> (w444:dbl)
            n143 = Divide(x=w444, y=w449) -> (x/y=w447:dbl)
            n144 = Multiply(x=2.0, y=w447) -> (x*y=w442:dbl)
            n145 = Compound Arithmetic op=ADD(w443, w442) -> (w441:dbl)
          }
          frame "External Source" {
          }
        }
        n146 = Divide(x=w403, y=w377) -> (x/y=w374:dbl)
        n147 = Divide(x=w377, y=w403) -> (x/y=w406:dbl)
        n148 = case shown="\"Relative Height\"" "Trigger Source" {
          selector: "Trigger Source" -> [w429 _]
          tunnel: [w429 T12."Absolute Height" ("Trigger Source")] -> w392
          frame Default {
          }
          frame "Relative Height" {
          }
        }
        n149 = Compound Arithmetic op=MULTIPLY(100.0 ("value"), w410, w406) -> (w409:dbl)
        n150 = Max & Min(x=w409, y=40.0 ("x")) -> (max(x,y)=w407:dbl)  [unwired: 1 out]
        n151 = Not(x="Fwd sweep") -> (.not. x?=w368:bool)
        n152 = Compound Arithmetic op=MULTIPLY(w374, w407, w378) -> (w404:dbl)
        n153 = Compound Arithmetic op=MULTIPLY(w378, w407, w400) -> (w405:dbl)
        n154 = xnode "Read/Write Control"("FPGA VI Reference In"=w370, "error in"=w372, "rmp.p.useIntHeightAsStart"="Fwd sweep") -> ("FPGA VI Reference Out"=w424:T18, "error out"=w425:errorcluster, "rmp.p.params"=w423:T22, "rmp.p.triggerParams"=w422:T23)
        n155 = Bundle By Name(cluster=w422, "rmp.p.triggerPositive"="Direction", "rmp.triggerSource"=w392, "rmp.p.triggerLevel"=w416) -> (w421:T23)
        n156 = Bundle By Name(cluster=w423, "rmp.p.upRate"=w404, "rmp.p.downRate"=w405, "rmp.p.startPos"=w364, "rmp.p.clockDec"=w407, "rmp.p.recordClockDec"="recordClockDec", "rmp.p.enableHDTPointRecord"=TRUE, "rmp.p.pull"=w368) -> (w415:T22)
        n157 = Bundle By Name(cluster=w367, "rmp.p.resetEndPos"=FALSE) -> (w360:T21)
        n158 = Bundle By Name(cluster=w367, "rmp.p.resetEndPos"=w368) -> (w369:T21)
        n159 = xnode "Read/Write Control"("FPGA VI Reference In"=w424, "error in"=w425, "rmp.p.params"=w415, "rmp.p.triggerParams"=w421, "rmp.p.action"=cluster{"rmp.p.start":bool, "rmp.p.stop":bool} {"rmp.p.start"=FALSE, "rmp.p.stop"=FALSE}, "rmp.p.reset"=w369) -> ("FPGA VI Reference Out"=w363:T18, "error out"=w358:errorcluster)
        n160 = property on="Channels" class="LstBox (strict)"() -> ("Value"=w387:i32[])  [unwired: 2 in, 2 out]
        n161 = Initialize Array(0.0 ("element"), w359) -> (w389:dbl[])
        n162 = Array Size(array=w387) -> (size(s)=w386:i32)
        n163 = flat-sequence {
          tunnel: w358 -> [w427]
          tunnel: [w427] -> w357
          frame #0 {
            n164 = Wait (ms)(milliseconds to wait=u32 30) -> ()  [unwired: 1 out]
          }
        }
        n165 = Bundle(cluster=cluster{dbl[], dbl[]} {[], []} ("output cluster"), w389, w389) -> (w388:cluster{dbl[], dbl[]})
        n166 = Multiply(x=2, y=w386) -> (x*y=w380:i32)
        n167 = xnode "Read/Write Control"("FPGA VI Reference In"=w363, "error in"=w357, "rmp.p.reset"=w360) -> ("FPGA VI Reference Out"=w362:T18, "error out"=w361:errorcluster)
        n168 = Initialize Array(w388, w380) -> (w385:cluster{dbl[], dbl[]}[])
        n169 = Add(x=w380, y=2) -> (x+y=w381:i32)
        n170 = Initialize Array(0.0 ("element"), w359, w381) -> (w382:dbl[][])
      }
      frame "ForceCurveFast.Start" {
        w457 = u32 0 ("Elements Remaining")
        w472 = 8  # Channels perBuffer
        w469 = 20 ("Timeout (ms)")
        w468 = u32 500000 ("Requested Depth")
        n171 = call "InitAndEmptyImageBuffer.vi"("Saving buffer"=enum16{"main", "aux"}."main", "error in (no error)"=w487, "Requested Depth"=w468, "Timeout (ms)"=w469, "Refnum in"=w461) -> ("error out"=w466:errorcluster, "Refnum Out"=w464:T18)  [unwired: 5 in]
        n172 = call "InitAndEmptyImageBuffer.vi"("Saving buffer"=enum16{"main", "aux"}."aux", "error in (no error)"=w466, "Requested Depth"=w468, "Timeout (ms)"=w469, "Refnum in"=w464) -> ("error out"=w465:errorcluster, "Refnum Out"=w463:T18)  [unwired: 5 in]
        n173 = xnode "Read/Write Control"("FPGA VI Reference In"=w463, "error in"=w465) -> ("FPGA VI Reference Out"=w482:T18, "error out"=w483:errorcluster, "rmp.p.action"=w481:cluster{"rmp.p.start":bool, "rmp.p.stop":bool})
        n174 = Bundle By Name(cluster=w481, "rmp.p.start"=TRUE) -> (w480:cluster{"rmp.p.start":bool, "rmp.p.stop":bool})
        n175 = xnode "Read/Write Control"("FPGA VI Reference In"=w482, "error in"=w483, "rmp.p.action"=w480) -> ("FPGA VI Reference Out"=w460:T18, "error out"=w455:errorcluster)
        n176 = flat-sequence {
          tunnel: w455 -> [w489]
          tunnel: [w489] -> w454
          frame #0 {
            n177 = Wait (ms)(milliseconds to wait=u32 10) -> ()  [unwired: 1 out]
          }
        }
        n178 = while {
          shift-right: [w497] -> _
          shift-left: w457 -> [w507]
          shift-right: [w505] -> _
          shift-left: w457 -> [w506]
          shift-right: [w504] -> w452
          shift-left: w460 -> [w491]
          tunnel: [w503] -> w458 mode=concatenating
          tunnel: [w502] -> w459 mode=concatenating
          tunnel: w454 -> [w499]
          tunnel: 100 ("Timeout (ms)") -> [w498]
          tunnel: 10 ("Timeout (ms)") -> [w492]
          stop <- w508 stop-if-true
          n179 = xnode "Invoke Method"("FPGA VI Reference In"=w491, "error in"=w499, "Number of Elements"=w507, "Timeout (ms)"=w498) -> ("error out"=w496:errorcluster, "Data"=w502:fxp<+/-,18,1>[], "Elements Remaining"=w497:u32)  [unwired: 1 out]
          n180 = xnode "Invoke Method"("FPGA VI Reference In"=w491, "Number of Elements"=w506, "Timeout (ms)"=w492) -> ("error out"=w494:errorcluster, "Data"=w503:fxp<+/-,18,1>[], "Elements Remaining"=w505:u32)  [unwired: 1 in, 1 out]
          n181 = Merge Errors(w496, w494) -> (w495:errorcluster)
          n182 = call <vilib>:"Clear Errors.vi"("error in (no error)"=w495) -> ("error out"=w493:errorcluster)  [unwired: 5 in, 1 out]
          n183 = xnode "Read/Write Control"("FPGA VI Reference In"=w491, "error in"=w493) -> ("FPGA VI Reference Out"=w504:T18, "rmp.s.running"=w510:bool)  [unwired: 1 out]
          n184 = property on="Stop" class="Bool (strict)"() -> ("Value"=w501:bool)  [unwired: 2 in, 2 out]
          n185 = Not(x=w510) -> (.not. x?=w509:bool)
          n186 = Compound Arithmetic op=OR(w509, w501) -> (w508:bool)
          n187 = Not(x=w508) -> (.not. x?=→"Ramping?":bool)
        }
        n188 = Array Size(array=w458) -> (size(s)=w475:i32)
        n189 = Array Size(array=w459) -> (size(s)=w478:i32)
        n190 = Quotient & Remainder(x=w478, y=w472) -> (floor(x/y)=w477:i32)  [unwired: 1 out]
        n191 = Quotient & Remainder(x=w475, y=w472) -> (floor(x/y)=w476:i32)  [unwired: 1 out]
        n192 = Reshape Array(w459, w477, w472) -> (w474:fxp<+/-,18,1>[][])
        n193 = Reshape Array(w458, w476, w472) -> (w473:fxp<+/-,18,1>[][])
        n194 = Insert Into Array(array=w474, index (col)=w472, new element=w473) -> (w471:fxp<+/-,18,1>[][])  [unwired: 1 in]
      }
      frame "AfterForceCurve" {
        n195 = local read "Fwd sweep"() -> (w513:bool)
        n196 = case shown="False" w513 {
          tunnel: [w526 w557] -> w525
          tunnel: [w527 w558] -> w518
          tunnel: w517 -> [w549 w557]
          tunnel: w516 -> [w547 w558]
          tunnel: w515 -> [w536 _]
          tunnel: w514 -> [w533 _]
          frame False {
            w545 = TRUE ("doMove")
            n197 = local read "Trigger Source"() -> (w542:T7)
            n198 = property on="Start" class="DigNum (strict)"() -> ("Value"=w544:dbl)  [unwired: 2 in, 2 out]
            n199 = Divide(x=w544, y=w536) -> (x/y=w535:dbl)
            n200 = local read "Dec"() -> (w531:u16)
            n201 = Multiply(x=w535, y=2.0) -> (x*y=w539:dbl)
            n202 = Equal?(x=w542, y=T7."Relative Height" ("Trigger Source")) -> (x = y?=w532:bool)
            n203 = Add(x=w533, y=w539) -> (x+y=w540:dbl)
            n204 = Select(t=w540, s=w532, f=w539) -> (s? t:f=w538:dbl)
            n205 = Reciprocal(x=w531) -> (1/x=w543:dbl)
            n206 = xnode "Read/Write Control"("FPGA VI Reference In"=w547, "error in"=w549) -> ("FPGA VI Reference Out"=w546:T18, "error out"=w548:errorcluster, "fb.mot.p.params"=w537:T20)
            n207 = Bundle By Name(cluster=w537, "integratorTarget"=w538, "clocks.decimation"=w531, "clocks.inverseDecimation"=w543, "enableManualMotion"=w545, "doMove"=w545) -> (w528:T20)
            n208 = xnode "Read/Write Control"("FPGA VI Reference In"=w546, "error in"=w548, "fb.mot.p.params"=w528) -> ("FPGA VI Reference Out"=w530:T18, "error out"=w529:errorcluster)
            n209 = while {
              tunnel: w530 -> [w556]
              tunnel: [w555] -> w527
              tunnel: w529 -> [w553]
              tunnel: [w554] -> w526
              stop <- w552 stop-if-true
              n210 = xnode "Read/Write Control"("FPGA VI Reference In"=w556, "error in"=w553) -> ("FPGA VI Reference Out"=w555:T18, "error out"=w554:errorcluster, "fb.mot.s.running"=w551:bool)
              n211 = Wait (ms)(milliseconds to wait=u32 20) -> ()  [unwired: 1 out]
              n212 = Not(x=w551) -> (.not. x?=w552:bool)
            }
          }
          frame True {
          }
        }
        n213 = xnode "Read/Write Control"("FPGA VI Reference In"=w518, "error in"=w525, "rmp.p.action"=cluster{"rmp.p.start":bool, "rmp.p.stop":bool} {"rmp.p.start"=FALSE, "rmp.p.stop"=FALSE}, "flt.bypassPI"=FALSE) -> ("FPGA VI Reference Out"=w519:T18, "error out"=w520:errorcluster)
      }
      frame "Data.Process" {
        n214 = local read "Trigger Source"() -> (w579:T7)
        n215 = Bundle(cluster=T13 {"Range Z"=0.0, "Parameters"={"Start"=0.0, "Distance"=0.0, "Points"=0.0, "Fwd"=0.0, "Bwd"=0.0, "Pause"=0.0}, "Trigger Source"=enum."Absolute Height"} ("InputParameters"), "Range Z"=w574, "Parameters"="Parameters", "Trigger Source"=w579) -> (w578:T13)
        n216 = call "ForceCurveDecimated.vi"("SaveArrayIn"=w573, "AcquiredChannels"="Channels", "error in (no error)"=w585, "InputParameters"=w578, "Data"=w582, "GraphIn"=w576) -> ("error out"=w570:errorcluster, "Fail"=w560:bool, "PointsMax"=w569:i32, "GraphOut"=w575:cluster{dbl[], "Decimated Array":dbl[]}[], "SaveArrayOut"=w572:dbl[][])  [unwired: 1 in]
        n217 = Number To Decimal String(number=w569) -> (decimal integer string=w566:string)  [unwired: 1 in]
        n218 = Search and Replace String(input string="Should be << to #", search string="#" ("regular expression"), replace string=w566) -> (result string=w565:string)  [unwired: 5 in, 3 out]
        n219 = Select(t=w565, s=w560, f="Number of decimated points") -> (s? t:f=w564:string)
        n220 = Select(t=u32 16711680 ("Color Box"), s=w560, f=u32 0 ("Color Box")) -> (s? t:f=w559:u32)
        n221 = property on="Points" class="DigNum (strict)"("TipStrip"=w564, "NumText.TextColor"=w559) -> ()  [unwired: 2 in, 2 out]
      }
      frame "GraphFast.Update" {
        w589 = FALSE
        w592 = 1 ("disabled index (col)")
        w590 = 0 ("disabled index (col)")
        w601 = u8 2 ("X Scale.Scale Fit")
        n222 = property on="ChannelDisplay" class="Ring (strict)"() -> ("Strings []"=w624:string[])  [unwired: 2 in, 2 out]
        n223 = local read "Parameters"() -> (w602:T4)
        n224 = Multiply(x="ChannelDisplay", y=u16 2) -> (x*y=w614:u16)
        n225 = Index Array(array=w624, index="ChannelDisplay") -> (element=w621:string)
        n226 = Increment(x=w614) -> (x+1=w616:u16)
        n227 = Index Array(array=w617, index #1=w614, index #2=w616) -> (element #1=w610:cluster{dbl[], "Decimated Array":dbl[]}, element #2=w609:cluster{dbl[], "Decimated Array":dbl[]})
        n228 = Concatenate Strings(w621, " (V)" ("Y Scale.Unit Label.Text")) -> (w620:string)
        n229 = Unbundle By Name(w602) -> ("Points"=w599:dbl)
        n230 = Build Array(w610, w609) -> (→"ForceCurves":cluster{dbl[], "Decimated Array":dbl[]}[])
        n231 = Decrement(x=w599) -> (x-1=w591:dbl)
        n232 = Index Array(array=w600, index (row) #1=w590, index (col) #1=w590, index (row) #2=w591, index (col) #2=w592, index (row) #3=w591, index (col) #3=w590, index (row) #4=w590, index (col) #4=w592) -> (element #1=w598:dbl, element #2=w597:dbl, element #3=w596:dbl, element #4=w595:dbl)
        n233 = Max & Min(x=w598, y=w597) -> (min(x,y)=w594:dbl)  [unwired: 1 out]
        n234 = Max & Min(x=w596, y=w595) -> (max(x,y)=w593:dbl)  [unwired: 1 out]
        n235 = Max & Min(x=w594, y=w593) -> (max(x,y)=w587:dbl, min(x,y)=w586:dbl)
        n236 = property on="ForceCurves" class="XYGraph (strict)"("YScale.NameLbl.Text"=w620, "XScale.Flipped"=w589, "XScale.Maximum"=w587, "XScale.Minimum"=w586, "XScale.ScaleFit"=w601) -> ()  [unwired: 2 in, 2 out]
        n237 = property on="ChannelDisplay2" class="Ring (strict)"() -> ("Strings []"=w625:string[])  [unwired: 2 in, 2 out]
        n238 = Multiply(x="ChannelDisplay2", y=u16 2) -> (x*y=w611:u16)
        n239 = Index Array(array=w625, index="ChannelDisplay2") -> (element=w619:string)
        n240 = Increment(x=w611) -> (x+1=w615:u16)
        n241 = Concatenate Strings(w619, " (V)" ("Y Scale.Unit Label.Text")) -> (w618:string)
        n242 = Index Array(array=w617, index #1=w611, index #2=w615) -> (element #1=w607:cluster{dbl[], "Decimated Array":dbl[]}, element #2=w606:cluster{dbl[], "Decimated Array":dbl[]})
        n243 = property on="ForceCurves 2" class="XYGraph (strict)"("YScale.NameLbl.Text"=w618, "XScale.Flipped"=w589, "XScale.Maximum"=w587, "XScale.Minimum"=w586, "XScale.ScaleFit"=w601) -> ()  [unwired: 2 in, 2 out]
        n244 = Build Array(w607, w606) -> (→"ForceCurves 2":cluster{dbl[], "Decimated Array":dbl[]}[])
      }
      frame "ScanSpeed.Lock" {
        n245 = Variant To Data(error in=w645, type=TRUE, Variant=w644) -> (data=w634:bool, error out=w642:errorcluster)
        n246 = Select(t=T11."Disabled and Grayed Out" ("Disabled"), s=w634, f=T11."Enabled" ("Disabled")) -> (s? t:f=w639:T11)
        n247 = property on="Bwd" class="DigNum (strict)"(error in=w642, "DisabledEnum"=w639) -> (error out=w633:errorcluster)  [unwired: 1 in, 1 out]
        n248 = property on="Bwd" class="DigNum (strict)"(error in=w633) -> (error out=w632:errorcluster, "Value"=w631:dbl)  [unwired: 1 in, 1 out]
        n249 = property on="Fwd" class="DigNum (strict)"(error in=w632) -> (error out=w638:errorcluster, "Value"=w636:dbl)  [unwired: 1 in, 1 out]
        n250 = Select(t=w636, s=w634, f=w631) -> (s? t:f=w635:dbl)
        n251 = property on="Bwd" class="DigNum (strict)"(error in=w638, "Val(Sgnl)"=w635) -> (error out=w637:errorcluster)  [unwired: 1 in, 1 out]
      }
      frame "TriggerSource.Update" {
        n252 = Variant To Data(error in=w662, type=T7."Absolute Height" ("NewVal"), Variant=w660) -> (data=w659:T7, error out=w661:errorcluster)
        n253 = case shown="\"Absolute Height\"" w659 {
          tunnel: w665 -> [_ _ _ _]
          tunnel: ["Distance" ("Caption.Text") "Fb Signal" ("Caption.Text") "Position" ("Caption.Text") "Trigger" ("Caption.Text")] -> w664
          tunnel: ["%#.3pm" ("Format String") "%#.3pV" ("Format String") "%#.3pm" ("Format String") "%#.3pV" ("Format String")] -> w656
          frame "Relative Height" {
          }
          frame "Process Variable", Default {
          }
          frame "Absolute Height" {
          }
          frame "External Source" {
          }
        }
        n254 = property on="Level" class="DigNum (strict)"(error in=w661, "Caption.Text"=w664, "FormatString"=w656) -> (error out=w663:errorcluster)  [unwired: 1 in, 1 out]
      }
      frame "Save" {
        w676 = "\t"
        w680 = "\n"
        n255 = property on="Parameters" class="Clust (strict)"() -> ("Controls[]"=w709:refnum<vi>[])  [unwired: 2 in, 2 out]
        n256 = Unbundle By Name("Saving") -> ("Path"=w693:path, "Name"=w683:string, "#"=w686:i64)
        n257 = Get Date/Time In Seconds() -> (seconds since 1Jan1904=w720:timestamp)
        n258 = property on="Channels" class="LstBox (strict)"() -> ("Item Names"=w704:string[])  [unwired: 2 in, 2 out]
        n259 = local read "Channels"() -> (w694:i32[])
        n260 = Format Date/Time String(time format string (%c)="%H-%M-%S", seconds (now)=w720) -> (date/time string=w719:string)  [unwired: 1 in]
        n261 = for {
          tunnel: w709 -> [w755] mode=indexing
          tunnel: [w750] -> w703 mode=indexing
          workers-P: _ -> [_]
          w747 = "\t"
          n262 = property class="Ctl"(reference=w755) -> ("Label.Text"=w751:string, "Value"=w754:variant)  [unwired: 1 in, 2 out]
          n263 = Variant To Data(type=0.0, Variant=w754) -> (data=w749:dbl)  [unwired: 1 in, 1 out]
          n264 = Format Value(format string="%.3e", value (0)=w749) -> (output string=w752:string)  [unwired: 1 in]
          n265 = Concatenate Strings(w751, w747, w752, w747) -> (w750:string)
        }
        n266 = Concatenate Strings("Position (m)", w676, w676) -> (w677:string)
        n267 = Concatenate Strings("Ramp_", w719) -> (w684:string)
        n268 = Empty String/Path?(string/path=w683) -> (empty?=w688:bool)
        n269 = for {
          tunnel: w704 -> [w740]
          tunnel: w694 -> [w741] mode=indexing
          shift-right: [w738] -> w696
          shift-left: w677 -> [w739]
          w736 = "\t"
          n270 = Index Array(array=w740, index=w741) -> (element=w737:string)
          n271 = Concatenate Strings(w739, w736, w737, w736, w736, w736) -> (w738:string)
        }
        n272 = Select(t=w684, s=w688, f=w683) -> (s? t:f=w706:string)
        n273 = Number To Decimal String(number=w686) -> (decimal integer string=w721:string)  [unwired: 1 in]
        n274 = Concatenate Strings(w706, "_" ("string"), w721) -> (w689:string)
        n275 = call "SaveCreatePath.vi"("Exp Folder"="<date>_exp<#>", "ExperimentNumber"=u32 0, "BaseFolder"=w693) -> ("appended path"=w690:path)  [unwired: 7 in, 1 out]
        n276 = Build Path(base path=w690, name or relative path=w689) -> (appended path=w716:path)
        n277 = Open/Create/Replace File(file path (use dialog)=w716, error in=w724, operation (0:open)=T14."create") -> (refnum out=w710:refnum<file>, error out=w725:errorcluster)  [unwired: 3 in, 1 out]
        n278 = Write to Text File(file (use dialog)=w710, text=w703, error in=w725) -> (refnum out=w702:refnum<file>, error out=w727:errorcluster)  [unwired: 1 in, 1 out]
        n279 = Write to Text File(file (use dialog)=w702, text=w696, error in=w727) -> (refnum out=w699:refnum<file>, error out=w697:errorcluster)  [unwired: 1 in, 1 out]
        n280 = Array Size(array=w694) -> (size(s)=w695:i32)
        n281 = Increment(x=w695) -> (x+1=w679:i32)
        n282 = for {
          N: w679 -> [_]
          shift-right: [w733] -> w682
          shift-left: w680 -> [w732]
          w731 = "\t"
          n283 = Concatenate Strings(w732, "Fwd" ("string"), w731, w731, "Bwd" ("string"), w731, w731) -> (w733:string)
        }
        n284 = Select(t=w686, s=w688, f=i64 -1 ("#")) -> (s? t:f=w685:i64)
        n285 = Concatenate Strings(w682, w680) -> (w681:string)
        n286 = Write to Text File(file (use dialog)=w699, text=w681, error in=w697) -> (refnum out=w698:refnum<file>, error out=w729:errorcluster)  [unwired: 1 in, 1 out]
        n287 = Array To Spreadsheet String(array=w728, 3:"%.4e" ("format string")) -> (spreadsheet string=w713:string)  [unwired: 1 in]
        n288 = Write to Text File(file (use dialog)=w698, text=w713, error in=w729) -> (refnum out=w715:refnum<file>, error out=w712:errorcluster)  [unwired: 1 in, 1 out]
        n289 = Close File(refnum=w715, error in=w712) -> (error out=w708:errorcluster)  [unwired: 1 out]
        n290 = case shown="No Error" w708 {
          tunnel: "Saving" -> [w746 _]
          tunnel: w685 -> [w744 _]
          frame No Error {
            n291 = Increment(x=w744) -> (x+1=w745:i64)
            n292 = Bundle By Name(cluster=w746, "#"=w745) -> (w743:T6)
            n293 = property on="Save" class="Bool (strict)"("Value"=FALSE) -> ()  [unwired: 2 in, 2 out]
            n294 = local write "Saving"(w743) -> ()
          }
          frame Error {
          }
        }
      }
      frame "Exit" {
        n295 = Release Queue(queue=w767, error in (no error)=w764) -> (error out=w765:errorcluster)  [unwired: 1 in, 2 out]
        n296 = Merge Errors(w765) -> (w763:errorcluster)
      }
      frame "Feedback.Reenable" {
        n297 = disable-structure shown="Enabled" {
          disable-tunnel: w783 -> [w808 w814]
          disable-tunnel: w782 -> [w807 w813]
          disable-tunnel: [w803 w811] -> w781
          disable-tunnel: w780 -> [w799 _]
          disable-tunnel: [w798 w815] -> w779
          disable-tunnel: [w797 w812] -> w778
          frame Disabled {
            n298 = Multiply(x=0.05 ("y"), y=w799) -> (x*y=w801:dbl)
            n299 = Subtract(x=w799, y=w801) -> (x-y=w802:dbl)
            n300 = Increment(x=w802) -> (x+1=w796:dbl)
            n301 = xnode "Read/Write Control"("FPGA VI Reference In"=w808, "error in"=w807) -> ("FPGA VI Reference Out"=w806:T18, "error out"=w805:errorcluster, "fb.mot.p.params"=w804:T20)
            n302 = Bundle By Name(cluster=w804, "integratorTarget"=w796, "enableManualMotion"=TRUE, "doMove"=TRUE) -> (w803:T20)
            n303 = xnode "Read/Write Control"("FPGA VI Reference In"=w806, "error in"=w805, "fb.mot.p.params"=w803) -> ("FPGA VI Reference Out"=w798:T18, "error out"=w797:errorcluster)
          }
          frame Enabled {
            n304 = xnode "Read/Write Control"("FPGA VI Reference In"=w814, "error in"=w813) -> ("FPGA VI Reference Out"=w815:T18, "error out"=w812:errorcluster, "fb.mot.p.params"=w811:T20)
          }
        }
        n305 = while {
          tunnel: w778 -> [w821]
          tunnel: w779 -> [w820]
          tunnel: [w819] -> w784
          tunnel: [w818] -> w787
          stop <- w817 stop-if-true
          n306 = xnode "Read/Write Control"("FPGA VI Reference In"=w820, "error in"=w821) -> ("FPGA VI Reference Out"=w819:T18, "error out"=w818:errorcluster, "fb.mot.s.running"=w816:bool)
          n307 = Not(x=w816) -> (.not. x?=w817:bool)
        }
        n308 = Bundle By Name(cluster=w781, "enableManualMotion"=FALSE, "doMove"=FALSE) -> (w773:T20)
        n309 = xnode "Read/Write Control"("FPGA VI Reference In"=w784, "error in"=w787, "fb.mot.p.params"=w773, "fb.p.enable"=TRUE ("enableFeedback")) -> ("FPGA VI Reference Out"=w771:T18, "error out"=w770:errorcluster)
        n310 = while {
          tunnel: w770 -> [w795]
          tunnel: w771 -> [w794]
          tunnel: [w793] -> w769
          tunnel: [w792] -> w768
          stop <- w791 stop-if-true
          n311 = xnode "Read/Write Control"("FPGA VI Reference In"=w794, "error in"=w795) -> ("FPGA VI Reference Out"=w793:T18, "error out"=w792:errorcluster, "fb.p.enable"=w791:bool)
          n312 = property on="Pause" class="DigNum (strict)"() -> ("Value"=w789:dbl)  [unwired: 2 in, 2 out]
          n313 = To Unsigned Long Integer(number=w789) -> (unsigned 32bit integer=w790:u32)
          n314 = Wait (ms)(milliseconds to wait=w790) -> ()  [unwired: 1 out]
        }
      }
      frame "SaveToImage" {
        w823 = refnum<vi> refnum  # Cluster
        w837 = TRUE ("Hide Grid")
        n315 = Variant To Data(error in=w858, type=refnum<vi> refnum ("CtlRef"), Variant=w856) -> (data=w827:refnum<vi>, error out=w828:errorcluster)
        n316 = property class="Bool"(reference=w827, error in=w828) -> (error out=w824:errorcluster, "Owner"=w822:refnum<vi>)  [unwired: 1 out]
        n317 = local read "Saving"() -> (w838:T6)
        n318 = Unbundle By Name(w838) -> ("Path"=w829:path, "Name"=w850:string, "#"=w863:i64)
        n319 = To More Specific Class(target class=w823, reference=w822, error in=w824) -> (specific class reference=w826:refnum<vi>, error out=w825:errorcluster)
        n320 = Get Date/Time In Seconds() -> (seconds since 1Jan1904=w844:timestamp)
        n321 = Format Date/Time String(time format string (%c)="%H-%M-%S", seconds (now)=w844) -> (date/time string=w842:string)  [unwired: 1 in]
        n322 = property class="Clust"(reference=w826, error in=w825) -> (error out=w854:errorcluster, "Label.Text"=w836:string)  [unwired: 1 out]
        n323 = Concatenate Strings("Ramp_", w842) -> (w848:string)
        n324 = Not Equal?(x=w850, y="") -> (x != y?=w847:bool)
        n325 = case shown="\"Palet1\"" w836 {
          tunnel: [w865 "" ("YScale.NameLbl.Text") w867] -> w835
          frame "Palet2" {
            n326 = property on="ForceCurves 2" class="XYGraph (strict)"() -> ("YScale.NameLbl.Text"=w865:string)  [unwired: 2 in, 2 out]
          }
          frame "Oops", Default {
          }
          frame "Palet1" {
            n327 = property on="ForceCurves" class="XYGraph (strict)"() -> ("YScale.NameLbl.Text"=w867:string)  [unwired: 2 in, 2 out]
          }
        }
        n328 = Select(t=w850, s=w847, f=w848) -> (s? t:f=w846:string)
        n329 = Number To Decimal String(number=w863) -> (decimal integer string=w853:string)  [unwired: 1 in]
        n330 = Concatenate Strings(w846, "_" ("string"), w853, w835) -> (w852:string)
        n331 = call "SaveCreatePath.vi"("Exp Folder"="<date>_exp<#>", "ExperimentNumber"=u32 0, "BaseFolder"=w829) -> ("appended path"=w830:path)  [unwired: 7 in, 1 out]
        n332 = Build Path(base path=w830, name or relative path=w852) -> (appended path=w841:path)
        n333 = case shown="\"Palet1\"" w836 {
          tunnel: [w874 w875 w881] -> w857
          tunnel: w854 -> [w873 w875 _]
          tunnel: w841 -> [w872 _ w878]
          tunnel: enum32{"BMP", "EPS", "EMF", "PICT"}."BMP" ("File Type") -> [w871 _ w880]
          tunnel: enum32{"File", "Clipboard"}."File" ("Target") -> [w870 _ w879]
          tunnel: w837 -> [w869 _ w877]
          tunnel: w837 -> [w868 _ w876]
          frame "Palet2" {
            n334 = invoke on="ForceCurves 2" class="XYGraph (strict)" method="Export Image"(error in=w873, "FileType"=w871, "Target"=w870, "Path"=w872, "HideGrid"=w869, "Overwrite"=w868) -> (error out=w874:errorcluster)  [unwired: 2 in, 7 out]
          }
          frame Default {
          }
          frame "Palet1" {
            n335 = invoke on="ForceCurves" class="XYGraph (strict)" method="Export Image"("FileType"=w880, "Target"=w879, "Path"=w878, "HideGrid"=w877, "Overwrite"=w876) -> (error out=w881:errorcluster)  [unwired: 3 in, 7 out]
          }
        }
      }
      frame "Save.ChangeName" {
        n336 = property on="#" class="DigNum (strict)"(error in=w888, "Value"=i64 0) -> (error out=w887:errorcluster)  [unwired: 1 in, 1 out]
      }
      frame Default {
        n337 = Format Into String(format string="The message\"%s\" received in the gestion loop is not valid" ("Texte de message d'erreur inconnu"), w902) -> (resulting string=w899:string)  [unwired: 2 in, 1 out]
        n338 = call <vilib>:"Error Cluster From Error Code.vi"("error message (\"\")"=w899, "error code (0)"=1 ("code d'erreur (0)")) -> ("error out"=w900:errorcluster)  [unwired: 7 in]
      }
    }
  }
  n339 = while {
    tunnel: w8 -> [w910]
    tunnel: [w906] -> w7
    tunnel: [w905] -> _
    stop <- w908 stop-if-true
    n340 = event shown="[10] \"CalculateSlope\": Mouse Down" {
      selector: _ -> [_ _ _ _ _ _ _ _ _ _ _ _ _ _ _]
      dyn-events: [_ _ _ _ _ _ _ _ _ _ _ _ _ _ _] -> w905
      timeout: 200 -> [_ _ _ _ _ _ _ _ _ _ _ _ _ _ _]
      tunnel: [w929 _ _ _ _ _ _ _ _ _ _ _ _ _ _] -> w909
      tunnel: w910 -> [w924 w931 w935 w941 w944 w949 w953 w957 w962 w966 w976 w980 w985 w991 w996]
      tunnel: [w928 _ _ w939 _ w946 w950 _ w959 _ _ w977 _ w989 _] -> w906
      tunnel: [w927 w931 w934 w940 w943 w947 w952 w955 w961 w966 w976 w979 w984 w990 w995] -> w907
      event Panel Close? {
        w922 = TRUE ("Message prioritaire ? (F)")
        w929 = TRUE ("Rejeter ?")
        n341 = event-data() -> ()  [unwired: 1 in, 1 out]
        n342 = call "Enqueue Message.vi"("Prioritary message"=w922, "Data"=TRUE, "Message"="DataAcquisition.OpenClose", "Queue"=w924) -> ("Queue dup."=w930:refnum<queue>)  [unwired: 6 in, 1 out]
        n343 = call "Enqueue Message.vi"("Prioritary message"=w922, "Message"="Exit", "Queue"=w930) -> ("error out"=w928:errorcluster, "Queue dup."=w927:refnum<queue>)  [unwired: 7 in]
        n344 = event-data ("Event Filter Node")("Discard?"=w929) -> ()  [unwired: 1 in, 1 out]
      }
      event Timeout {
        n345 = event-data() -> ()  [unwired: 1 in, 3 out]
      }
      event "Trigger Source": Value Change {
        n346 = event-data() -> ("NewVal"=w933:T7)  [unwired: 1 in]
        n347 = call "Enqueue Message.vi"("Data"=w933, "Message"="TriggerSource.Update" ("QueueName"), "Queue"=w935) -> ("Queue dup."=w934:refnum<queue>)  [unwired: 7 in, 1 out]
      }
      event "Actions.Sweeps", "Actions.Loop": Value Change; "Actions.Play", "Actions.Stop": Mouse Down {
        n348 = event-data() -> ("CtlRef"=w937:refnum<vi>)  [unwired: 1 in]
        n349 = call "Enqueue Message.vi"("Prioritary message"=TRUE, "Data"=w937, "Message"="Action.Send", "Queue"=w941) -> ("error out"=w939:errorcluster, "Queue dup."=w940:refnum<queue>)  [unwired: 6 in]
      }
      event "Parameters.Distance": Value Change {
        n350 = event-data() -> ()  [unwired: 1 in, 6 out]
        n351 = call "Enqueue Message.vi"("Message"="Panel.Initialize", "Queue"=w944) -> ("Queue dup."=w943:refnum<queue>)  [unwired: 8 in, 1 out]
      }
      event "ChannelDisplay", "ChannelDisplay2": Value Change {
        n352 = event-data() -> ("NewVal"=w945:u16)  [unwired: 1 in]
        n353 = call "Enqueue Message.vi"("Data"=w945, "Message"="GraphFast.Update", "Queue"=w949) -> ("error out"=w946:errorcluster, "Queue dup."=w947:refnum<queue>)  [unwired: 7 in]
      }
      event "Saving.Save": Mouse Down {
        n354 = event-data() -> ()  [unwired: 1 in, 1 out]
        n355 = call "Enqueue Message.vi"("Message"="Save", "Queue"=w953) -> ("error out"=w950:errorcluster, "Queue dup."=w952:refnum<queue>)  [unwired: 8 in]
      }
      event "Saving.Name", "Saving.Path": Value Change {
        n356 = event-data() -> ("CtlRef"=w954:refnum<vi>)  [unwired: 1 in]
        n357 = call "Enqueue Message.vi"("Data"=w954, "Message"="Save.ChangeName", "Queue"=w957) -> ("Queue dup."=w955:refnum<queue>)  [unwired: 7 in, 1 out]
      }
      event "Channels": Value Change {
        n358 = event-data() -> ("NewVal"=w958:i32[])  [unwired: 1 in]
        n359 = call "Enqueue Message.vi"("Data"=w958, "Message"="Channel.Select", "Queue"=w962) -> ("error out"=w959:errorcluster, "Queue dup."=w961:refnum<queue>)  [unwired: 7 in]
      }
      event "ForceCurves": Cursor Move {
        n360 = event-data() -> ("CursIdx"=w963:i32, "CursRef"=w965:refnum<vi>)  [unwired: 1 in]
        n361 = property class="Curs"(reference=w965) -> ("Cursor Position"=w964:T24)  [unwired: 1 in, 2 out]
        n362 = case shown="1" w963 {
          tunnel: w964 -> [w967 w968]
          frame 0, Default {
            "A" <- w967
          }
          frame 1 {
            "B" <- w968
          }
        }
      }
      event "CalculateSlope": Mouse Down {
        n363 = event-data() -> ()  [unwired: 1 in, 1 out]
        n364 = property on="A" class="Clust (strict)"() -> ("Value"=w975:cluster{"Y":dbl, "X":dbl})  [unwired: 2 in, 2 out]
        n365 = property on="B" class="Clust (strict)"() -> ("Value"=w974:cluster{"Y":dbl, "X":dbl})  [unwired: 2 in, 2 out]
        n366 = Subtract(x=w975, y=w974) -> (x-y=w973:cluster{"Y":dbl, "X":dbl})
        n367 = Unbundle By Name(w973) -> ("Y"=w972:dbl, "X"=w971:dbl)
        n368 = Divide(x=w972, y=w971) -> (x/y=w970:dbl)
        n369 = Absolute Value(x=w970) -> (abs(x)=→"1/Slope":dbl)
      }
      event "ForceCurves", "ForceCurves 2": Value Change {
        n370 = event-data() -> ()  [unwired: 1 in, 1 out]
        n371 = call "Enqueue Message.vi"("Message"="Graph.Update", "Queue"=w980) -> ("error out"=w977:errorcluster, "Queue dup."=w979:refnum<queue>)  [unwired: 8 in]
      }
      event "Palet1.Save", "Palet2.Save": Mouse Down {
        n372 = event-data() -> ("CtlRef"=w982:refnum<vi>)  [unwired: 1 in]
        n373 = To Variant(anything=w982) -> (Variant=w981:variant)
        n374 = call "Enqueue Message.vi"("Data"=w981, "Message"="SaveToImage", "Queue"=w985) -> ("Queue dup."=w984:refnum<queue>)  [unwired: 7 in, 1 out]
      }
      event "LockSpeed": Value Change {
        n375 = event-data() -> ("NewVal"=w987:bool)  [unwired: 1 in]
        n376 = call "Enqueue Message.vi"("Prioritary message"=TRUE, "Data"=w987, "Message"="ScanSpeed.Lock", "Queue"=w991) -> ("error out"=w989:errorcluster, "Queue dup."=w990:refnum<queue>)  [unwired: 6 in]
      }
      event "Parameters.Fwd": Value Change {
        n377 = event-data() -> ()  [unwired: 1 in, 3 out]
        n378 = local read "LockSpeed"() -> (w993:bool)
        n379 = To Variant(anything=w993) -> (Variant=w992:variant)
        n380 = call "Enqueue Message.vi"("Data"=w992, "Message"="ScanSpeed.Lock", "Queue"=w996) -> ("Queue dup."=w995:refnum<queue>)  [unwired: 7 in, 1 out]
      }
    }
    n381 = case shown="Error" w906 {
      selector: w906 -> [_ w916]
      tunnel: [w911 TRUE ("Rejeter ?")] -> w908
      tunnel: w909 -> [w911 _]
      tunnel: w907 -> [_ w921]
      frame No Error {
      }
      frame Error {
        w912 = TRUE ("Message prioritaire ? (F)")
        n382 = call "Enqueue Message.vi"("Prioritary message"=w912, "error in"=w916, "Data"=FALSE, "Message"="DataAcquisition.OpenClose", "Queue"=w921) -> ("error out"=w914:errorcluster, "Queue dup."=w915:refnum<queue>)  [unwired: 5 in]
        n383 = call "Enqueue Message.vi"("Prioritary message"=w912, "error in"=w914, "Data"=TRUE, "Message"="Exit", "Queue"=w915) -> ()  [unwired: 5 in, 2 out]
      }
    }
  }
  n384 = Merge Errors(w7, w11) -> (w13:errorcluster)
  n385 = disable-structure shown="Disabled" {
    disable-tunnel: w13 -> [w999 w1000]
    disable-tunnel: [w998 w1000] -> w12
    disable-tunnel: w10 -> [w997 _]
    frame Disabled {
      n386 = xnode "Close FPGA VI Reference"("FPGA VI Reference In"=w997, "error in"=w999) -> ("error out"=w998:errorcluster)
    }
    frame Enabled {
    }
  }
  n387 = call <vilib>:"Simple Error Handler.vi"("error in (no error)"=w12) -> ()  [unwired: 4 in, 5 out]
